vi "Set Host.vi"(8 "error in (no error)":errorcluster, 10 "Host":string, 11 "Network Config in":refnum<class "Network Config.lvclass">) -> (0 "error out":errorcluster, 3 "Network Config out":refnum<class "Network Config.lvclass">)   [LabVIEW 2020, in "Examples.lvlib" / "Network Config.lvclass"]
uses:
  Network Config.lvclass
  Network Config.lvclass/Network Config.ctl
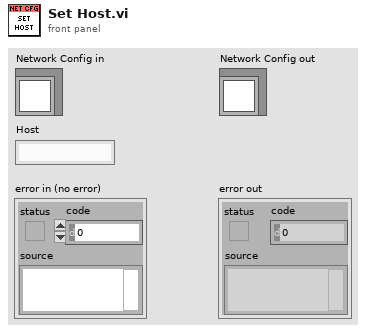
[diagram p1: front panel]
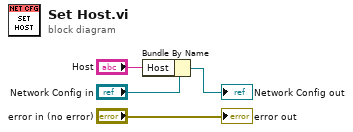
[diagram p0: block diagram]
diagram:
  n1 = Bundle By Name(cluster="Network Config in", "Host"="Host") -> (→"Network Config out":refnum<class "Network Config.lvclass">)
  "error out" <- "error in (no error)"
